vi "Data to Pedals Status.vi"(1 "Data":u8[](array[numeric]) format="%b") -> (0 "\"Pedals\" Status":T1 {"Acceleration pedal" scale=0.0..100.0 scale format="%.0f%%"; "Break pedal" scale=0.0..100.0 scale format="%.0f%%"})   [LabVIEW 2016]
uses:
  Pedals Status.ctl
panel:
  out "double precision float":dbl
  out "Data[1]":u8
  out "Data[0]":u8
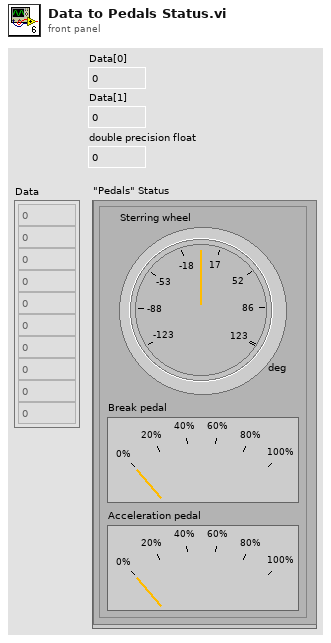
[diagram p1: front panel]
types:
  T1 = typedef "Pedals Status.ctl" = cluster{"Acceleration pedal":dbl, "Break pedal":dbl, "Sterring wheel":dbl[unit]}
  T2 = cluster{"Data[0]":u8, "Data[1]":u8, "Data[2]":u8, "Data[3]":u8, "Data[4]":u8, "Data[5]":u8, "Data[6]":u8, "Data[7]":u8, "Data[8]":u8}
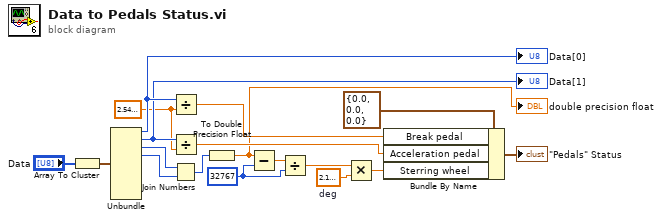
[diagram p0: block diagram]
diagram:
  w3 = dbl[unit] 2.1467549799530254  # deg
  w5 = u16 32767
  w8 = sgl 2.55 ("y")
  n1 = Array To Cluster(array="Data") -> (cluster=w15:T2)
  n2 = Unbundle(w15) -> ("Data[0]"=w12:u8, "Data[1]"=w11:u8, "Data[2]"=w14:u8, "Data[3]"=w13:u8)  [unwired: 5 out]
  "Data[0]" <- w12
  "Data[1]" <- w11
  n3 = Divide(x=w12, y=w8) -> (x/y=w10:sgl)
  n4 = Divide(x=w11, y=w8) -> (x/y=w9:sgl)
  n5 = Join Numbers(hi=w14, lo=w13) -> ((hi.lo)=w7:u16)
  n6 = To Double Precision Float(number=w7) -> (double precision float=w2:dbl)
  "double precision float" <- w2
  n7 = Subtract(x=w2, y=w5) -> (x-y=w6:dbl)
  n8 = Divide(x=w6, y=w5) -> (x/y=w4:dbl)
  n9 = Multiply(x=w4, y=w3) -> (x*y=w1:dbl[unit])
  n10 = Bundle By Name(cluster=T1 {"Acceleration pedal"=0.0, "Break pedal"=0.0, "Sterring wheel"=0.0} ("\"Pedals\" Status"), "Break pedal"=w10, "Acceleration pedal"=w9, "Sterring wheel"=w1) -> (→"\"Pedals\" Status":T1)
